vi "CN Enable image&Fit.vi"(8 "error in (no error)":errorcluster, 10 "CN Pic Ref":refnum<vi>[](array[refnum]), 11 "CN image":T1) -> (0 "error out":errorcluster, 3 "CN image out":T1)   [LabVIEW 2014]
uses:
  <vilib>/picture/picture.llb/imagedata.ctl
  Type'def/CN Config Ctr.ctl
  Type'def/CN image Ctr.ctl
panel:
  out "CN Enable":refnum<vi>[](array[refnum])
  out "Tab":T4(array[ring])
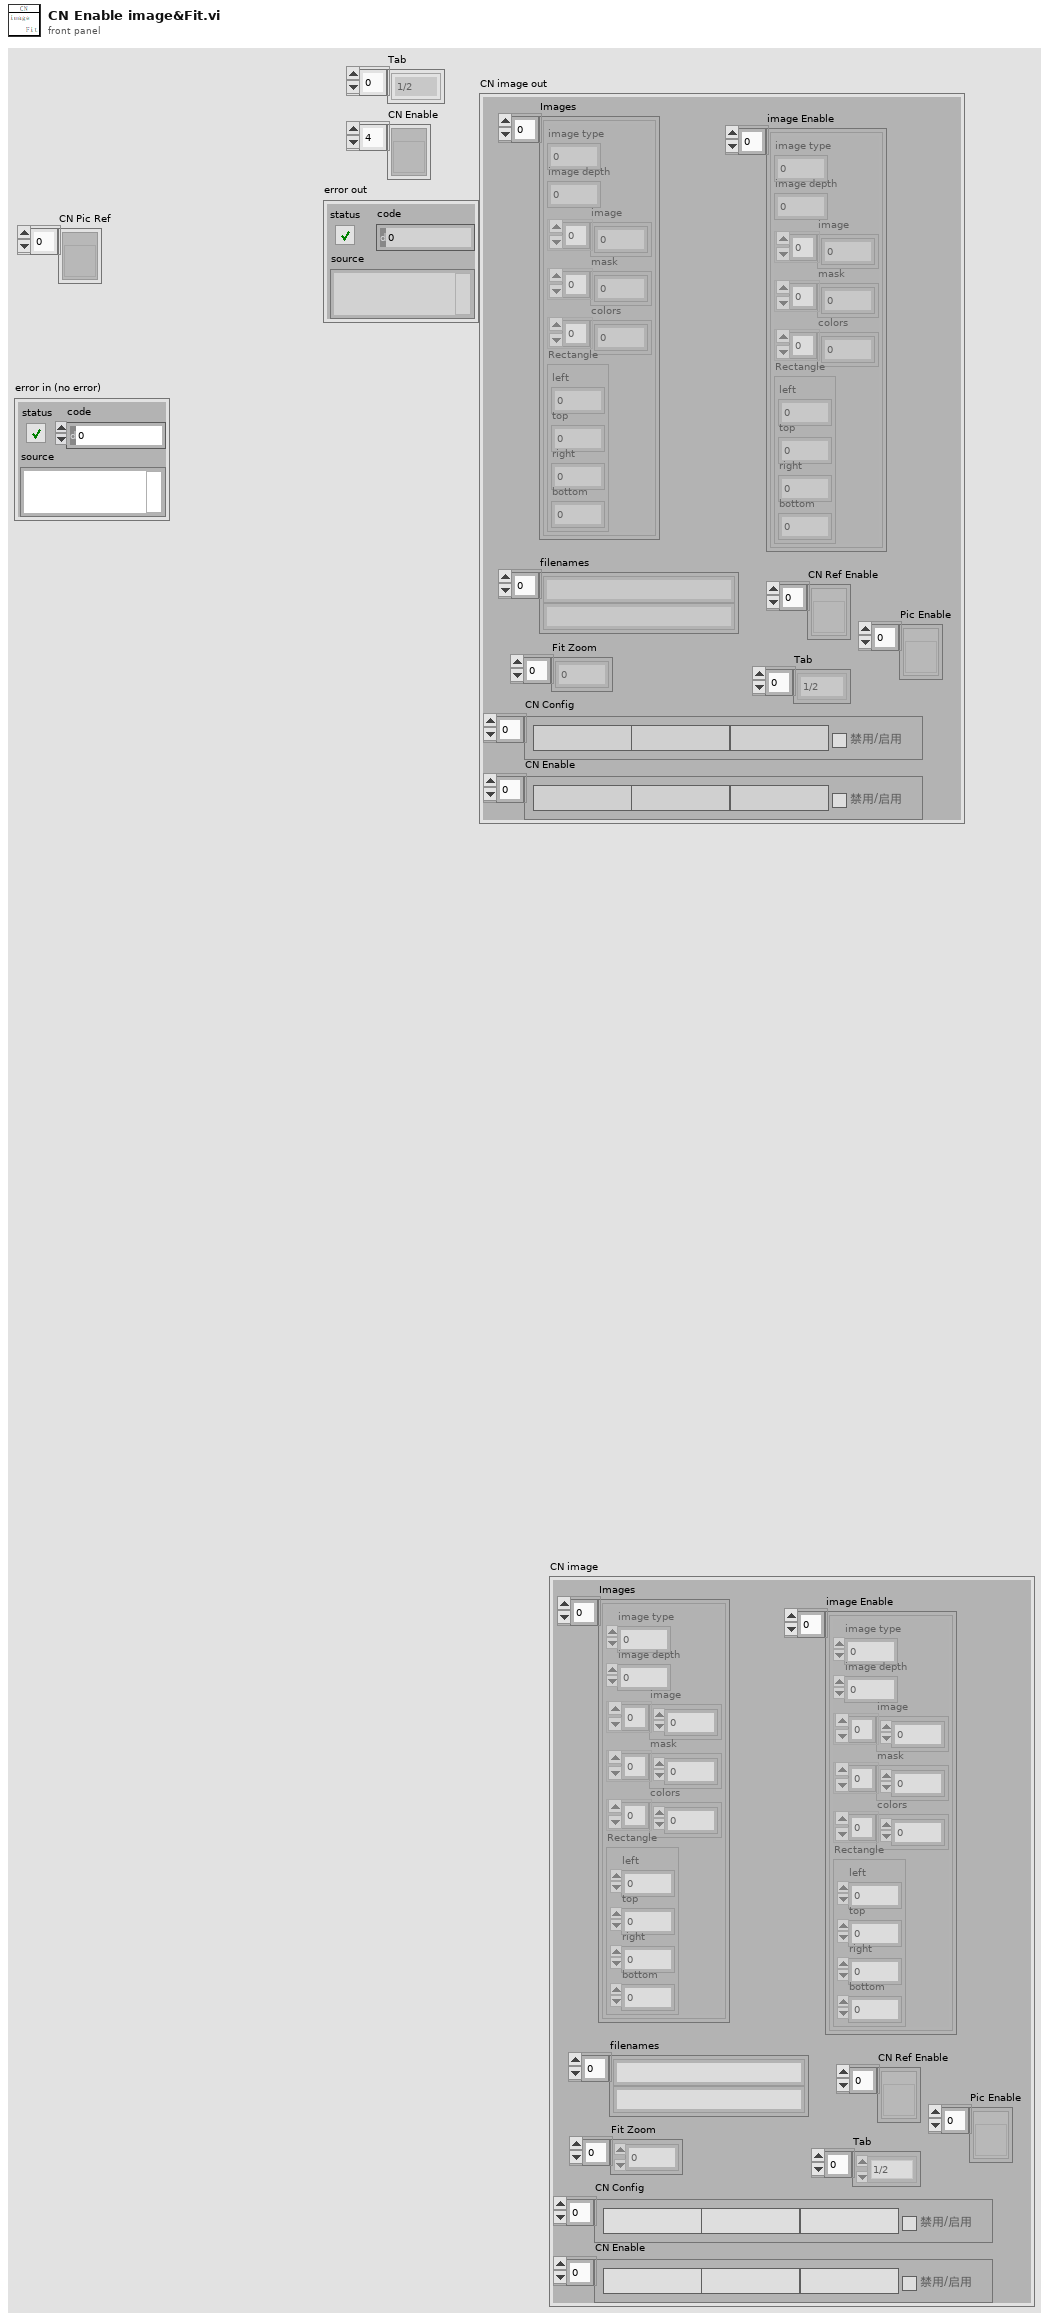
[diagram p1: front panel]
types:
  T1 = typedef "CN image Ctr.ctl" = cluster{"Images":T2[], "filenames":string[], "Fit Zoom":dbl[], "CN Config":T3[], "CN Enable":T3[], "image Enable":T2[], "CN Ref Enable":refnum<vi>[], "Tab ":enum32{"1/2", "1/3", "1/4", "1/5", "2/5", "3/5"}[], "Pic Enable":refnum<vi>[]}
  T2 = typedef "imagedata.ctl" = cluster{"image type":i32, "image depth":i32, "image":u8[], "mask":u8[], "colors":u32[], "Rectangle":cluster{"left":i16, "top":i16, "right":i16, "bottom":i16}}
  T3 = typedef "CN Config Ctr.ctl" = cluster{"Model":string, "Pic_Name":string, "CarName":string, "En/Disable":bool}
  T4 = enum32{"1/2", "1/3", "1/4", "1/5", "2/5", "3/5"}[]
  T5 = typedef "LVBoundsTypeDef.ctl" = cluster{"Width":u32, "Height":u32}
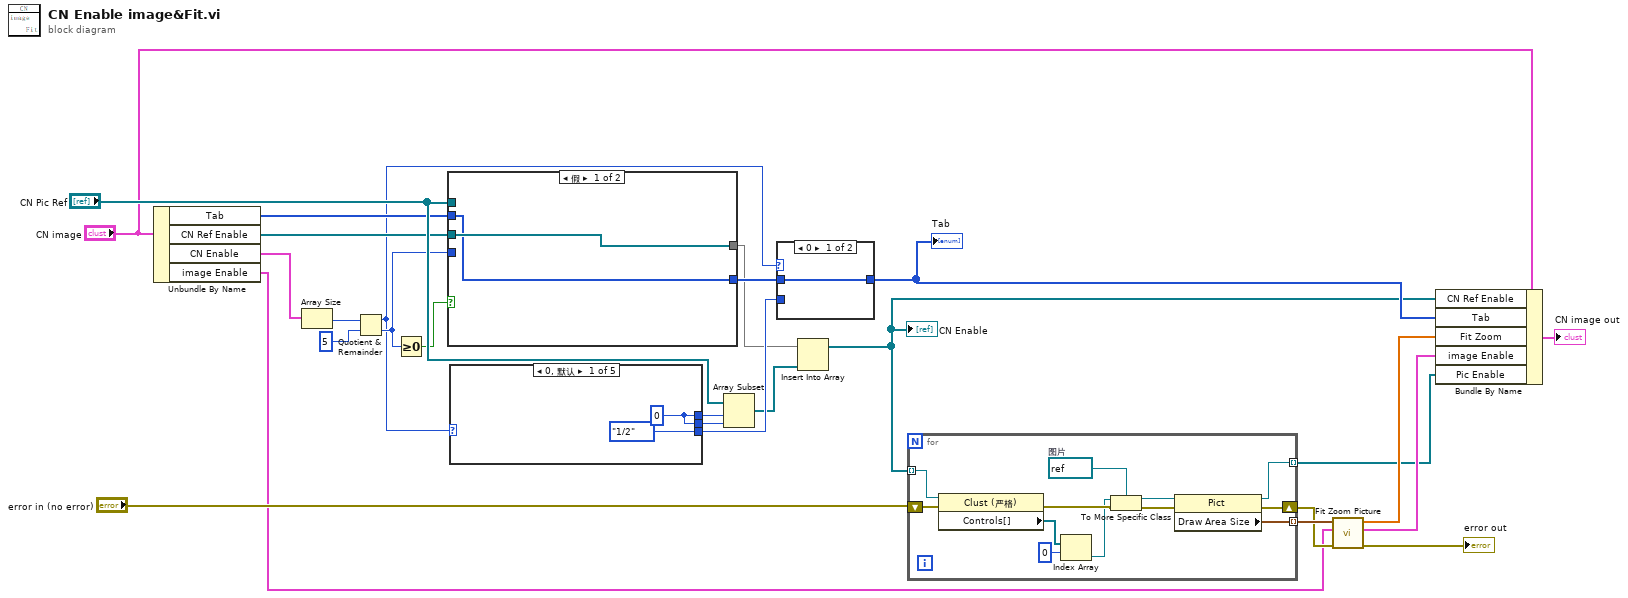
[diagram p0: block diagram]
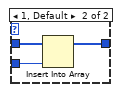
[diagram p2: hidden frame]
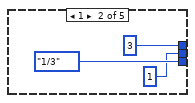
[diagram p3: hidden frame]
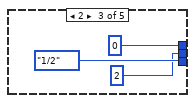
[diagram p4: hidden frame]
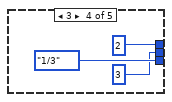
[diagram p5: hidden frame]
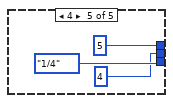
[diagram p6: hidden frame]
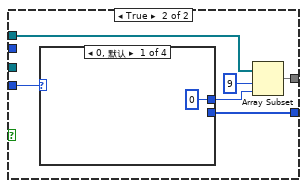
[diagram p7: hidden frame]
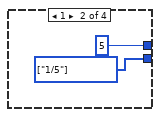
[diagram p8: hidden frame]
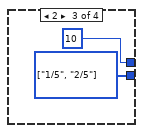
[diagram p9: hidden frame]
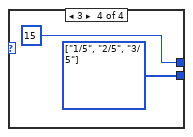
[diagram p10: hidden frame]
diagram:
  n1 = Unbundle By Name("CN image") -> ("Tab"=w13:T4, "CN Ref Enable"=w14:refnum<vi>[], "CN Enable"=w25:T3[], "image Enable"=w9:T2[])
  n2 = Array Size(array=w25) -> (size(s)=w24:i32)
  n3 = Quotient & Remainder(x=w24, y=5) -> (x-y*floor(x/y)=w1:i32, floor(x/y)=w21:i32)
  n4 = Greater Or Equal To 0?(x=w21) -> (x >= 0?=w22:bool)
  n5 = case shown="假" w22 {
    tunnel: w21 -> [_ w35]
    tunnel: [w28 w34] -> w20
    tunnel: "CN Pic Ref" -> [_ w33]
    tunnel: [w29 w30] -> w16
    tunnel: w14 -> [w29 _]
    tunnel: w13 -> [w28 _]
    frame False {
    }
    frame True {
      n6 = case shown="0, 默认" w35 {
        tunnel: [_ w38 w40 w42] -> w34
        tunnel: [0 ("length") 5 ("length") 10 ("length") 15 ("length")] -> w31
        frame 0, Default {
        }
        frame 1 {
          w38 = T4 [enum."1/5"] items=["1/2", "1/3", "1/4", "1/5", "2/5", "3/5"]
        }
        frame 2 {
          w40 = T4 [enum."1/5", enum."2/5"] items=["1/2", "1/3", "1/4", "1/5", "2/5", "3/5"]
        }
        frame 3 {
          w42 = T4 [enum."1/5", enum."2/5", enum."3/5"] items=["1/2", "1/3", "1/4", "1/5", "2/5", "3/5"]
        }
      }
      n7 = Array Subset(array=w33, index=9, length=w31) -> (w30:refnum<vi>[])
    }
  }
  n8 = case shown="0, 默认" w1 {
    tunnel: [enum32{"1/2", "1/3", "1/4", "1/5", "2/5", "3/5"}."1/2" ("Tab CN") enum32{"1/2", "1/3", "1/4", "1/5", "2/5", "3/5"}."1/3" ("Tab CN") enum32{"1/2", "1/3", "1/4", "1/5", "2/5", "3/5"}."1/2" ("Tab CN") enum32{"1/2", "1/3", "1/4", "1/5", "2/5", "3/5"}."1/3" ("Tab CN") enum32{"1/2", "1/3", "1/4", "1/5", "2/5", "3/5"}."1/4" ("Tab CN")] -> w19
    tunnel: [w44 3 0 2 5] -> w18
    tunnel: [w44 1 2 3 4] -> w17
    frame 0, Default {
      w44 = 0
    }
    frame 1 {
    }
    frame 2 {
    }
    frame 3 {
    }
    frame 4 {
    }
  }
  n9 = Array Subset(array="CN Pic Ref", index=w18, length=w17) -> (w15:refnum<vi>[])
  n10 = case shown="0" w1 {
    tunnel: w20 -> [w57 w60]
    tunnel: w19 -> [_ w59]
    tunnel: [w57 w58] -> w6
    frame 0 {
    }
    frame 1, Default {
      n11 = Insert Into Array(array=w60, new element=w59) -> (w58:T4)  [unwired: 1 in]
    }
  }
  "Tab" <- w6
  n12 = Insert Into Array(array=w16, new element=w15) -> (w5:refnum<vi>[])  [unwired: 1 in]
  "CN Enable" <- w5
  n13 = for {
    tunnel: w5 -> [w71] mode=indexing
    tunnel: [w63] -> w12 mode=indexing
    shift-right: [w62] -> w11
    shift-left: "error in (no error)" -> [w72]
    tunnel: [w61] -> w4 mode=indexing
    w65 = refnum<vi> refnum  # 图片
    n14 = property class="Clust (严格)"(reference=w71, error in=w72) -> (error out=w68:errorcluster, "Controls[]"=w70:refnum<vi>[])  [unwired: 1 out]
    n15 = Index Array(array=w70, index=0) -> (element=w67:refnum<vi>)
    n16 = To More Specific Class(target class=w65, reference=w67, error in=w68) -> (specific class reference=w64:refnum<vi>, error out=w66:errorcluster)
    n17 = property class="Pict"(reference=w64, error in=w66) -> (reference out=w61:refnum<vi>, error out=w62:errorcluster, "Draw Area Size"=w63:T5)
  }
  n18 = call "Fit Zoom Picture.vi"("error in (no error)"=w11, "Images"=w9, "Draw Area Size"=w12) -> ("error out"=→"error out":errorcluster, "Images out"=w8:T2[], "Fit Zoom"=w7:dbl[])  [unwired: 6 in]
  n19 = Bundle By Name(cluster="CN image", "CN Ref Enable"=w5, "Tab"=w6, "Fit Zoom"=w7, "image Enable"=w8, "Pic Enable"=w4) -> (→"CN image out":T1)
